vi "Change Set Temperature 9620.vi"(8 "error in (no error)":errorcluster, 10 "Temperture Setpoint":dbl, 11 "VISA resource name":refnum<visa-resource-name>="COM3") -> (0 "error out":errorcluster, 3 "VISA resource name out":refnum<visa-resource-name>)   [LabVIEW 2017]
doc: "This changes the temperature setpoint. If you want to query the setpoint after this, make sure there is a 0.2 s delay (according to manual)."
panel:
  out "Command string":string="S"
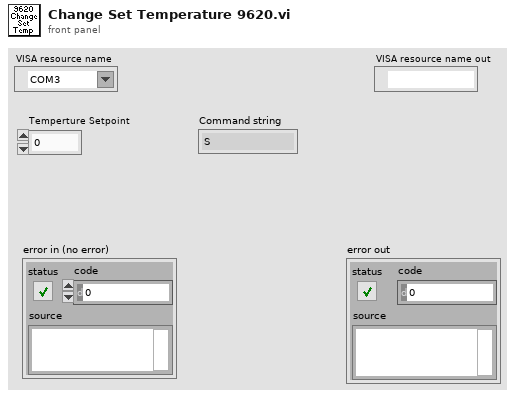
[diagram p1: front panel]
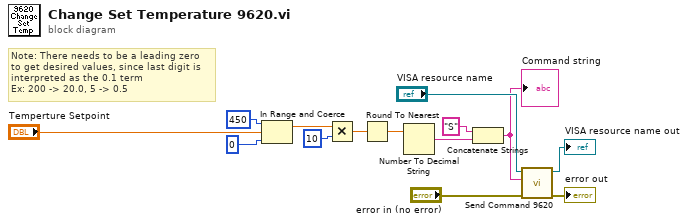
[diagram p0: block diagram]
diagram:
  # "Note: There needs to be a leading zero \nto get desired values, since last digit is\ninterpreted as the 0.1 term\nEx: 200 -> 20.0, 5 -> 0.5"
  n1 = In Range and Coerce(upper limit=450, x="Temperture Setpoint", lower limit=0) -> (coerced(x)=w7:dbl)  [unwired: 1 out]
  n2 = Multiply(x=w7, y=10) -> (x*y=w4:dbl)
  n3 = Round To Nearest(number=w4) -> (nearest integer value=w3:dbl)
  n4 = Number To Decimal String(number=w3) -> (decimal integer string=w10:string)  [unwired: 1 in]
  n5 = Concatenate Strings("S", w10) -> (w1:string)
  "Command string" <- w1
  n6 = call "Send Command 9620.vi"("error in (no error)"="error in (no error)", "command"=w1, "VISA resource name"="VISA resource name") -> ("error out"=→"error out":errorcluster, "VISA resource name out"=→"VISA resource name out":refnum<visa-resource-name>)  [unwired: 7 in]
